vi "Configure Session.vi"(8 "error in":errorcluster, 11 "Plugin in":refnum<class "PXIe-4113 DC Power Supply NI-DCPower Runtime Plugin PowerSupply.lvclass">) -> (0 "error out":errorcluster, 3 "Plugin out":refnum<class "PXIe-4113 DC Power Supply NI-DCPower Runtime Plugin PowerSupply.lvclass">)   [LabVIEW 2026, in "PXIe-4113 DC Power Supply NI-DCPower Runtime Plugin PowerSupply.lvlib" / "PXIe-4113 DC Power Supply NI-DCPower Runtime Plugin PowerSupply.lvclass"]
uses:
  PXIe-4113 DC Power Supply NI-DCPower Runtime Plugin PowerSupply.lvclass
  C:/Program Files/National Instruments/LabVIEW 2026/vi.lib/FlexLogger/SDK/PluginSDK.lvlibp/PEFClasses/SDK/Plugin/Plugin.lvclass
  PXIe-4113 DC Power Supply NI-DCPower Runtime Plugin PowerSupply.lvclass/PXIe-4113 DC Power Supply NI-DCPower Runtime Plugin PowerSupply.ctl
  <vilib>/FlexLogger/SDK/PluginSDK.lvlibp/PEFClasses/SDK/Plugin/ParameterAccess/Read String.vi
  <vilib>/FlexLogger/SDK/PluginSDK.lvlibp/PEFClasses/SDK/Plugin/ParameterAccess/Read DBL.vi
  <vilib>/FlexLogger/SDK/PluginSDK.lvlibp/PEFClasses/SDK/Plugin/Plugin.lvclass
  C:/Program Files/National Instruments/LabVIEW 2026/vi.lib/FlexLogger/SDK/PluginSDK.lvlibp/PEFClasses/SDK/Processing Element/Processing Element.lvclass
  C:/Users/krael/OneDrive - Emerson/Documents/LabVIEW Projects/FlexLogger IO Plug-ins/PXIe-4113 DC Power Supply NI-DCPower Runtime Plugin PowerSupply/PXIe-4113 DC Power Supply NI-DCPower Runtime Plugin PowerSupply.lvclass
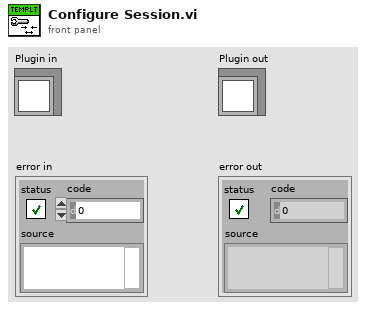
[diagram p1: front panel]
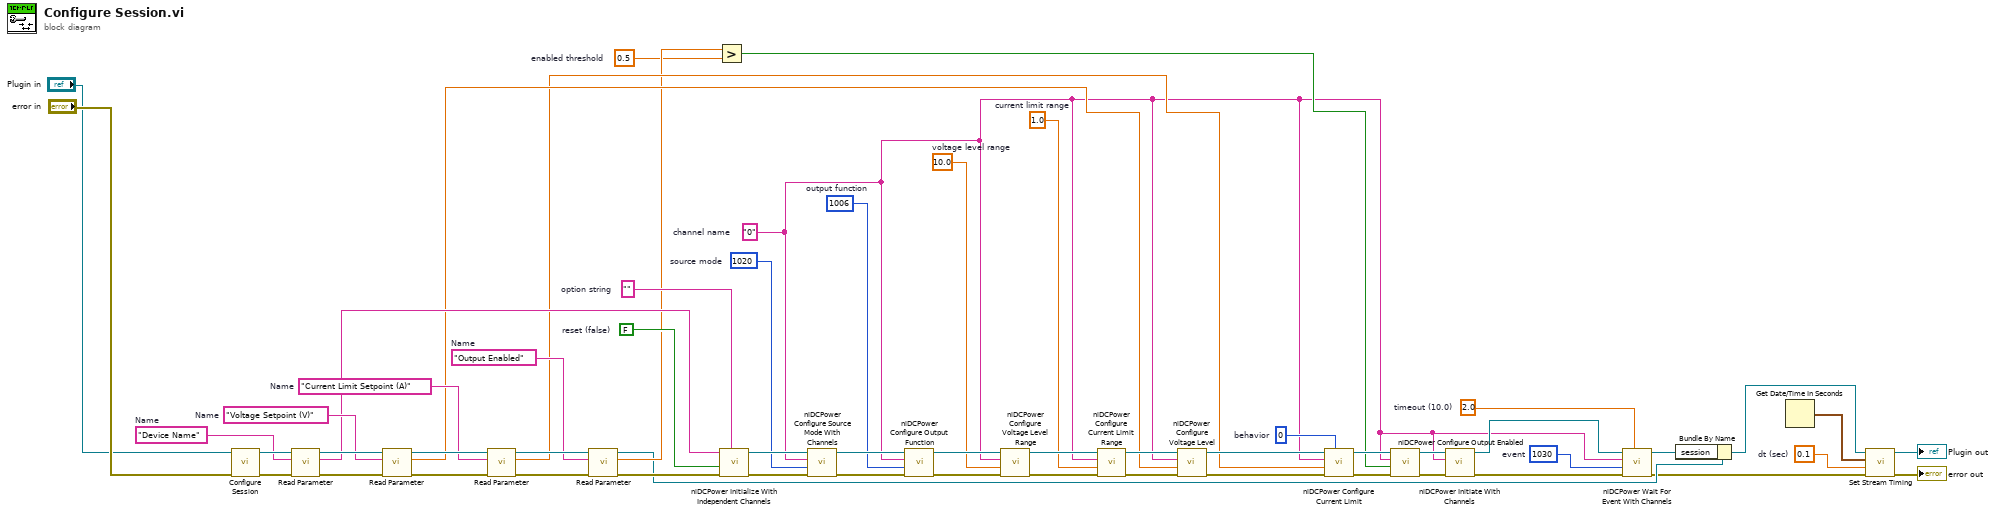
[diagram p0: block diagram]
diagram:
  w4 = 0.1  # dt (sec)
  w9 = 2.0  # timeout (10.0)
  w11 = 1030  # event
  w19 = 0.5  # enabled threshold
  w21 = 0  # behavior
  w29 = 1.0  # current limit range
  w32 = 10.0  # voltage level range
  w35 = 1006  # output function
  w38 = 1020  # source mode
  w40 = ""  # option string
  w42 = FALSE  # reset (false)
  w12 = "0"  # channel name
  w45 = "Output Enabled"  # Name
  w48 = "Current Limit Setpoint (A)"  # Name
  w51 = "Voltage Setpoint (V)"  # Name
  w54 = "Device Name"  # Name
  n1 = call-parent "Configure Session.vi"("error in (no error)"="error in", "Processing Element in"="Plugin in") -> ("error out"=w53:errorcluster, "Processing Element out"=w55:refnum<class "PXIe-4113 DC Power Supply NI-DCPower Runtime Plugin PowerSupply.lvclass">)  [unwired: 8 in]
  n2 = call-poly <vilib>:"Read Parameter.vi"("error in (no error)"=w53, "Name"=w54, "Plugin in"=w55) -> ("error out"=w50:errorcluster, "Value"=w43:string, "Plugin out"=w52:refnum<class "PXIe-4113 DC Power Supply NI-DCPower Runtime Plugin PowerSupply.lvclass">)  [unwired: 5 in, 1 out]
  n3 = call-poly <vilib>:"Read Parameter.vi"("error in (no error)"=w50, "Name"=w51, "Plugin in"=w52) -> ("error out"=w47:errorcluster, "Value"=w26:dbl, "Plugin out"=w49:refnum<class "PXIe-4113 DC Power Supply NI-DCPower Runtime Plugin PowerSupply.lvclass">)  [unwired: 5 in, 1 out]
  n4 = call-poly <vilib>:"Read Parameter.vi"("error in (no error)"=w47, "Name"=w48, "Plugin in"=w49) -> ("error out"=w44:errorcluster, "Value"=w23:dbl, "Plugin out"=w46:refnum<class "PXIe-4113 DC Power Supply NI-DCPower Runtime Plugin PowerSupply.lvclass">)  [unwired: 5 in, 1 out]
  n5 = call-poly <vilib>:"Read Parameter.vi"("error in (no error)"=w44, "Name"=w45, "Plugin in"=w46) -> ("error out"=w41:errorcluster, "Value"=w20:dbl, "Plugin out"=w7:refnum<class "PXIe-4113 DC Power Supply NI-DCPower Runtime Plugin PowerSupply.lvclass">)  [unwired: 5 in, 1 out]
  n6 = Greater?(x=w20, y=w19) -> (0:w17:bool)
  n7 = call <instrlib>:"niDCPower Initialize With Independent Channels.vi"("option string"=w40, "error in (no error)"=w41, "reset (false)"=w42, "resource name"=w43) -> ("error out"=w37:errorcluster, "instrument handle out"=w39:refnum<k15>)  [unwired: 6 in]
  n8 = call <instrlib>:"niDCPower Configure Source Mode With Channels.vi"("error in (no error)"=w37, "source mode"=w38, "channel name"=w12, "instrument handle"=w39) -> ("error out"=w34:errorcluster, "instrument handle out"=w36:refnum<k15>)  [unwired: 6 in]
  n9 = call <instrlib>:"niDCPower Configure Output Function.vi"("error in (no error)"=w34, "output function"=w35, "channel name"=w12, "instrument handle"=w36) -> ("error out"=w31:errorcluster, "instrument handle out"=w33:refnum<k15>)  [unwired: 6 in]
  n10 = call <instrlib>:"niDCPower Configure Voltage Level Range.vi"("error in (no error)"=w31, "voltage level range"=w32, "channel name"=w12, "instrument handle"=w33) -> ("error out"=w28:errorcluster, "instrument handle out"=w30:refnum<k15>)  [unwired: 6 in]
  n11 = call <instrlib>:"niDCPower Configure Current Limit Range.vi"("error in (no error)"=w28, "current limit range"=w29, "channel name"=w12, "instrument handle"=w30) -> ("error out"=w25:errorcluster, "instrument handle out"=w27:refnum<k15>)  [unwired: 6 in]
  n12 = call <instrlib>:"niDCPower Configure Voltage Level.vi"("error in (no error)"=w25, "voltage level"=w26, "channel name"=w12, "instrument handle"=w27) -> ("error out"=w22:errorcluster, "instrument handle out"=w24:refnum<k15>)  [unwired: 6 in]
  n13 = call <instrlib>:"niDCPower Configure Current Limit.vi"("behavior"=w21, "error in (no error)"=w22, "current limit"=w23, "channel name"=w12, "instrument handle"=w24) -> ("error out"=w16:errorcluster, "instrument handle out"=w18:refnum<k15>)  [unwired: 5 in]
  n14 = call <instrlib>:"niDCPower Configure Output Enabled.vi"("error in (no error)"=w16, "output enabled"=w17, "channel name"=w12, "instrument handle"=w18) -> ("error out"=w14:errorcluster, "instrument handle out"=w15:refnum<k15>)  [unwired: 6 in]
  n15 = call <instrlib>:"niDCPower Initiate With Channels.vi"("error in (no error)"=w14, "channel name"=w12, "instrument handle"=w15) -> ("error out"=w10:errorcluster, "instrument handle out"=w13:refnum<k15>)  [unwired: 7 in]
  n16 = call <instrlib>:"niDCPower Wait For Event With Channels.vi"("timeout (10.0)"=w9, "error in (no error)"=w10, "event"=w11, "channel name"=w12, "instrument handle"=w13) -> ("error out"=w3:errorcluster, "instrument handle out"=w8:refnum<k15>)  [unwired: 5 in]
  n17 = Bundle By Name(cluster=w7, "session"=w8) -> (w6:refnum<class "PXIe-4113 DC Power Supply NI-DCPower Runtime Plugin PowerSupply.lvclass">)
  n18 = Get Date/Time In Seconds() -> (seconds since 1Jan1904=w5:timestamp)
  n19 = call-dynamic "Set Stream Timing.vi"("error in (no error)"=w3, "dt(sec)"=w4, "Start Time"=w5, "Plugin in"=w6) -> ("error out"=→"error out":errorcluster, "Plugin out"=→"Plugin out":refnum<class "PXIe-4113 DC Power Supply NI-DCPower Runtime Plugin PowerSupply.lvclass">)  [unwired: 6 in]
